vi "Check Variables & Linked Channels Correspondence.vi"(7 "Command/Response Refnum in":T1 format="%.0x", 8 "error in (no error)":errorcluster, 9 "Variables in":string[](array[string]), 11 "Linked Channels in":cluster{"Variable Name":string, "GUID":string}[](array[cluster])) -> (0 "error out":errorcluster, 3 "Linked Channels out":T2[](array[typedef]))   [LabVIEW 2018, in "Instrument Addon Scripting API.lvlib"]
uses:
  Instrument Addon Scripting API.lvlib
  Addon/Addon Shared/Types/Linked Channel Cluster.ctl
  <vilib>/NI Veristand/Custom Device API/Custom Device Item Ref.ctl
  Addon/Addon Shared/Instrument Addon Shared.lvlib
  <vilib>/NI VeriStand/Custom Device API/Custom Device API.lvlib
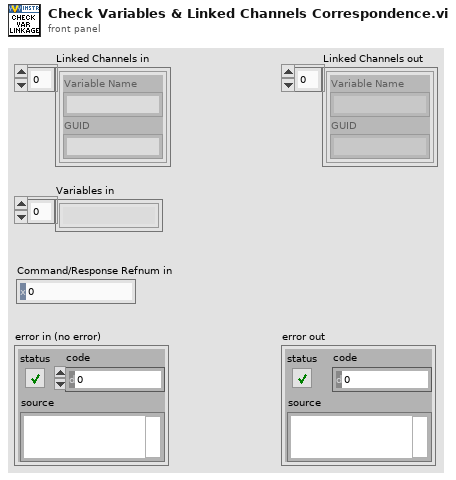
[diagram p1: front panel]
types:
  T1 = typedef "Custom Device API.lvlib/Custom Device Item Ref.ctl" = u64
  T2 = typedef "Instrument Addon Shared.lvlib/Linked Channel Cluster.ctl" = cluster{"Variable Name":string, "GUID":string}
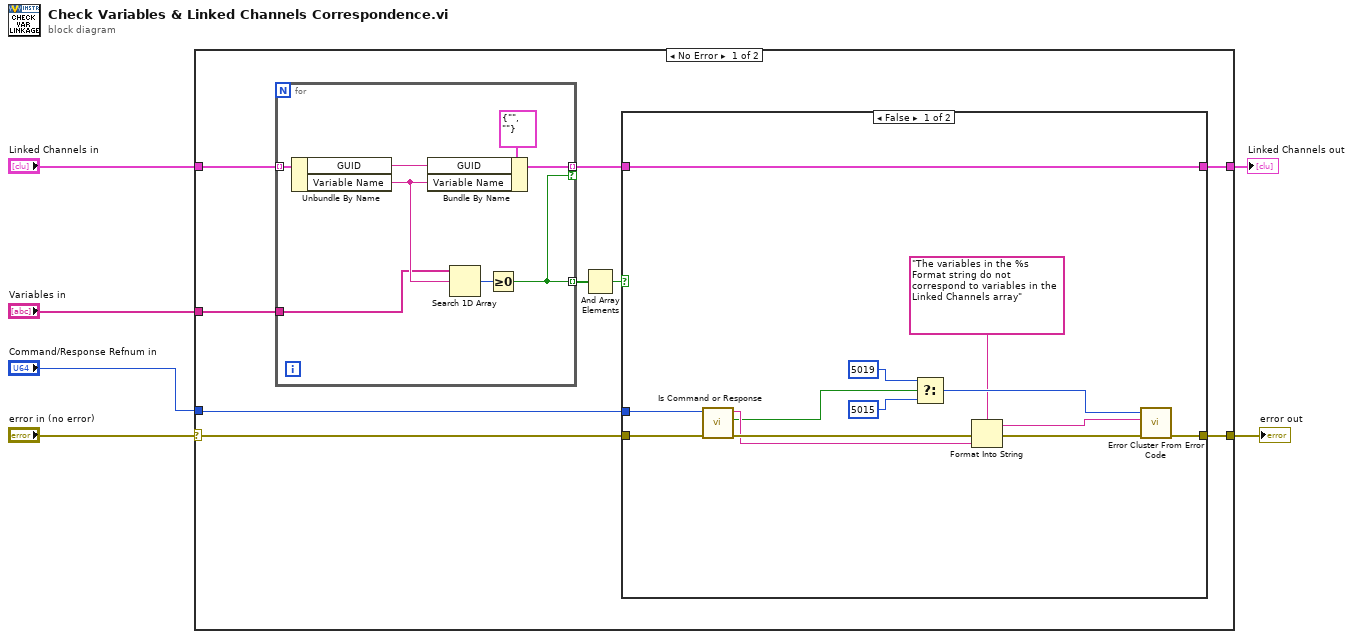
[diagram p0: block diagram]
diagram:
  n1 = case shown="No Error" "error in (no error)" {
    selector: "error in (no error)" -> [w8 w39]
    tunnel: "Linked Channels in" -> [w15 w40]
    tunnel: [w12 w39] -> w2
    tunnel: [w10 w40] -> w3
    tunnel: "Variables in" -> [w9 _]
    tunnel: "Command/Response Refnum in" -> [w7 _]
    frame No Error {
      n2 = for {
        tunnel: w15 -> [w37] mode=indexing
        tunnel: [w35] -> w11 mode=indexing if=w32
        tunnel: [w32] -> w14 mode=indexing
        tunnel: w9 -> [w31]
        n3 = Unbundle By Name(w37) -> ("GUID"=w36:string, "Variable Name"=w33:string)
        n4 = Bundle By Name(cluster=T2 {"Variable Name"="", "GUID"=""} ("Linked Channel"), "GUID"=w36, "Variable Name"=w33) -> (w35:T2)
        n5 = Search 1D Array(1D array=w31, element=w33) -> (index of element=w34:i32)  [unwired: 1 in]
        n6 = Greater Or Equal To 0?(x=w34) -> (x >= 0?=w32:bool)
      }
      n7 = And Array Elements(Boolean array=w14) -> (logical AND=w13:bool)
      n8 = case shown="False" w13 {
        tunnel: [w28 w29] -> w12
        tunnel: w11 -> [w27 w30]
        tunnel: [w27 w30] -> w10
        tunnel: w8 -> [w20 w29]
        tunnel: w7 -> [w19 _]
        frame False {
          n9 = call "Is Command or Response.vi"("error in (no error)"=w20, "Command/Response Refnum in"=w19) -> ("error out"=w18:errorcluster, "Is Command?"=w16:bool, "Command/Response out"=w17:string)  [unwired: 7 in]
          n10 = Select(t=5019 ("error code (0)"), s=w16, f=5015 ("error code (0)")) -> (s? t:f=w23:i32)
          n11 = Format Into String(format string="The variables in the %s Format string do not correspond to variables in the Linked Channels array" ("error message (\"\")"), error in=w18, w17) -> (resulting string=w21:string, error out=w24:errorcluster)  [unwired: 1 in]
          n12 = call <vilib>:"Error Cluster From Error Code.vi"("error in (no error)"=w24, "error message (\"\")"=w21, "error code (0)"=w23) -> ("error out"=w28:errorcluster)  [unwired: 6 in]
        }
        frame True {
        }
      }
    }
    frame Error {
    }
  }
  "Linked Channels out" <- w3
  "error out" <- w2
